vi "Setup Statically-Linked subWorkers.vi"(8 "error in":errorcluster, 11 "cRIO NI 9205 Demo in":refnum<class "cRIO NI 9205 Demo.lvclass">) -> (0 "error out":errorcluster, 3 "cRIO NI 9205 Demo out":refnum<class "cRIO NI 9205 Demo.lvclass">)   [LabVIEW 2017, in "cRIO NI 9205 Demo.lvclass"]
doc: "This VI performs a setup of all the statically-linked subWorkers that belong to the Worker that owns this VI. This VI must be called <b>before</b> any statically-linked subWorkers are called."
uses:
  cRIO NI 9205 Demo.lvclass
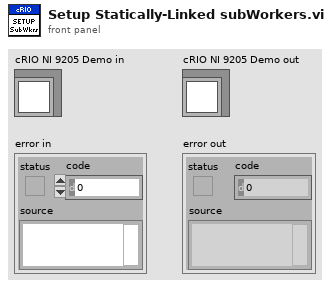
[diagram p1: front panel]
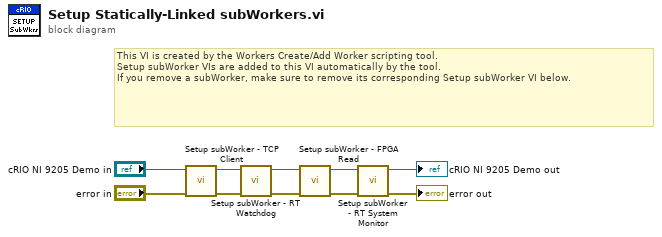
[diagram p0: block diagram]
diagram:
  # "This VI is created by the Workers Create/Add Worker scripting tool.\nSetup subWorker VIs are added to this VI automatically by the tool.\nIf you remove a subWorker, make sure to remove its corresponding Setup subWorker VI below."
  n1 = call "Setup subWorker - TCP Client.vi"("error in"="error in", "cRIO NI 9205 Demo in"="cRIO NI 9205 Demo in") -> ("error out"=w9:errorcluster, "cRIO NI 9205 Demo out"=w7:refnum<class "cRIO NI 9205 Demo.lvclass">)  [unwired: 8 in]
  n2 = call "Setup subWorker - RT Watchdog.vi"("error in"=w9, "cRIO NI 9205 Demo in"=w7) -> ("error out"=w4:errorcluster, "cRIO NI 9205 Demo out"=w5:refnum<class "cRIO NI 9205 Demo.lvclass">)  [unwired: 8 in]
  n3 = call "Setup subWorker - FPGA Read.vi"("error in"=w4, "cRIO NI 9205 Demo in"=w5) -> ("error out"=w6:errorcluster, "cRIO NI 9205 Demo out"=w2:refnum<class "cRIO NI 9205 Demo.lvclass">)  [unwired: 8 in]
  n4 = call "Setup subWorker - RT System Monitor.vi"("error in"=w6, "cRIO NI 9205 Demo in"=w2) -> ("error out"=→"error out":errorcluster, "cRIO NI 9205 Demo out"=→"cRIO NI 9205 Demo out":refnum<class "cRIO NI 9205 Demo.lvclass">)  [unwired: 8 in]
